vi "Read prueba.vi"(8 "error in (no error)":errorcluster) -> (0 "error out":errorcluster, 3 "num Prueba":string)   [LabVIEW 2020, in "Settings.lvlib"]
uses:
  Settings.lvlib
  <vilib>/drjdpowell/SQLite Library/SQL Connection/Open (path).vi
  <vilib>/drjdpowell/SQLite Library/SQL Connection/Open (string).vi
  <vilib>/AdvancedString/Path To Command Line String.vi
  <vilib>/drjdpowell/SQLite Library/SQL Connection/Execute SQL (1D String).vi
  <vilib>/drjdpowell/SQLite Library/SQL Connection/Connection.lvclass
  <vilib>/drjdpowell/SQLite Library/SQLite.lvlib
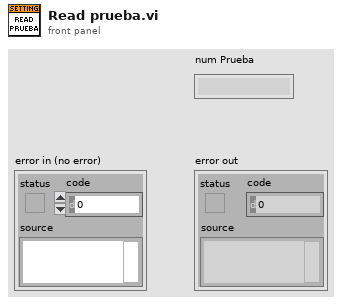
[diagram p1: front panel]
types:
  T1 = cluster{"Result Set[0]":string, "Result Set[1]":string, "Result Set[2]":string, "Result Set[3]":string, "Result Set[4]":string, "Result Set[5]":string, "Result Set[6]":string, "Result Set[7]":string, "Result Set[8]":string}
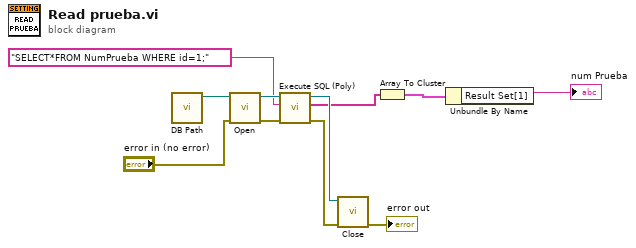
[diagram p0: block diagram]
diagram:
  n1 = call "DB Path.vi"() -> ("DB path"=w5:path)  [unwired: 11 in]
  n2 = call-poly <vilib>:"Open.vi"("error in (no error)"="error in (no error)", "db file"=w5) -> ("error out"=w11:errorcluster, "SQLite Connection"=w10:refnum<class "Connection.lvclass">)  [unwired: 8 in]
  n3 = call-poly <vilib>:"Execute SQL (Poly).vi"("error in (no error)"=w11, "SQL"="SELECT*FROM NumPrueba WHERE id=1;", "SQLite Connection in"=w10) -> ("error out"=w8:errorcluster, "Result Set"=w3:string[], "SQLite Connection"=w9:refnum<class "Connection.lvclass">)  [unwired: 5 in, 1 out]
  n4 = call-dynamic "Close.vi"("error in (no error)"=w8, "SQLite Connection in"=w9) -> ("error out"=→"error out":errorcluster)  [unwired: 9 in]
  n5 = Array To Cluster(array=w3) -> (cluster=w2:T1)
  n6 = Unbundle By Name(w2) -> ("Result Set[1]"=→"num Prueba":string)
